vi "SetOffsets.vi"(8 "error in (no error)":errorcluster, 9 "Y offset":i32, 10 "X offset":i32, 11 "FolloWin in":refnum<class "FolloWin.lvclass">) -> (0 "error out":errorcluster, 3 "FolloWin out":refnum<class "FolloWin.lvclass">)   [LabVIEW 2023, in "FolloWin.lvclass"]
doc: "Sets the X and Y distance between the cursor and the top right corner of the FolloWin"
uses:
  FolloWin.lvclass
  FolloWin.lvclass/FolloWin.ctl
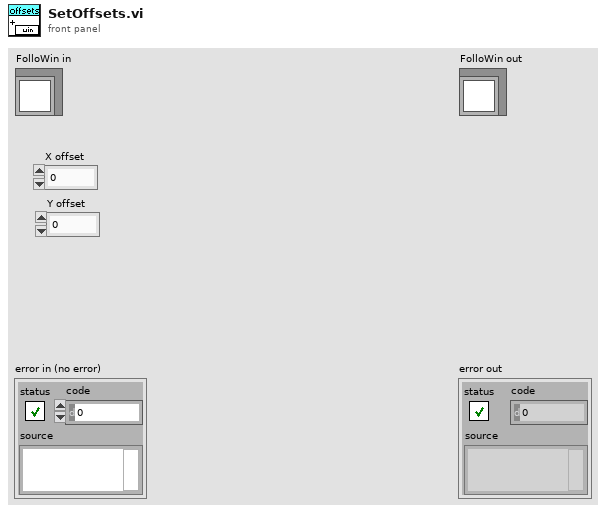
[diagram p1: front panel]
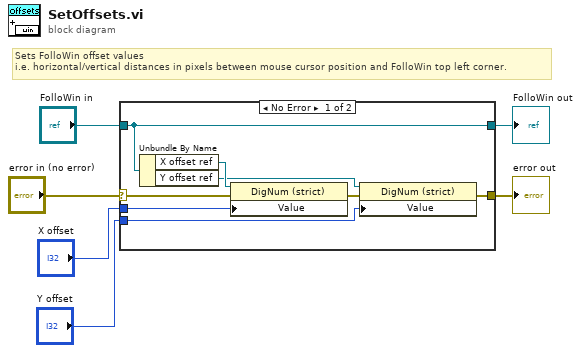
[diagram p0: block diagram]
diagram:
  # "Sets FolloWin offset values \ni.e. horizontal/vertical distances in pixels between mouse cursor position and FolloWin top left corner."
  n1 = case shown="No Error" "error in (no error)" {
    selector: "error in (no error)" -> [w9 w16]
    tunnel: [w10 w16] -> w5
    tunnel: [w14 w15] -> w3
    tunnel: "FolloWin in" -> [w14 w15]
    tunnel: "X offset" -> [w7 _]
    tunnel: "Y offset" -> [w8 _]
    frame No Error {
      n2 = Unbundle By Name(w14) -> ("X offset ref"=w13:refnum<vi>, "Y offset ref"=w12:refnum<vi>)
      n3 = property on="Property Node" class="DigNum (strict)"(reference=w13, error in=w9, "Value"=w7) -> (error out=w11:errorcluster)  [unwired: 1 out]
      n4 = property on="Property Node" class="DigNum (strict)"(reference=w12, error in=w11, "Value"=w8) -> (error out=w10:errorcluster)  [unwired: 1 out]
    }
    frame Error {
    }
  }
  "error out" <- w5
  "FolloWin out" <- w3
